vi "cummulative_threshold.vi"(0 "N":dbl[](array[numeric]), 5 "q(i)":dbl[](array[numeric]), 7 "Array 1 in":dbl[](array[numeric]), 9 "Array 2 in":dbl[](array[numeric]), 11 "Array 3 in":dbl[](array[numeric])) -> (4 "Cummulative Threshold Estimate [dB]":dbl=19.38227816273107, 8 "Array 1 out":dbl[](array[numeric]), 10 "Array 2 out":dbl[](array[numeric]), 15 "Array 3 out":dbl[](array[numeric]))   [LabVIEW 2022 SP3]
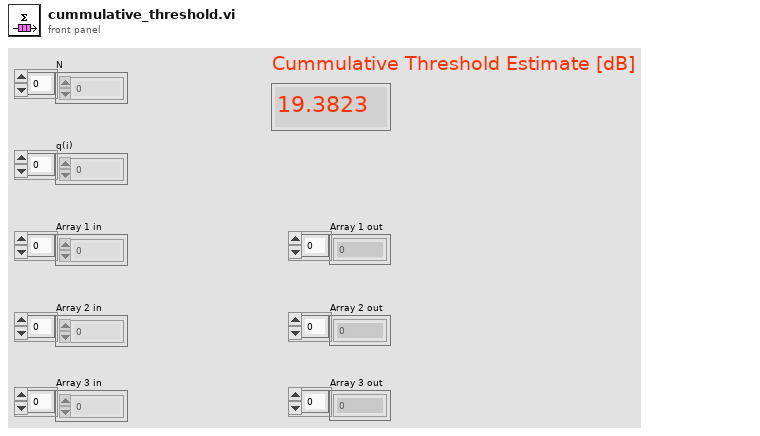
[diagram p1: front panel]
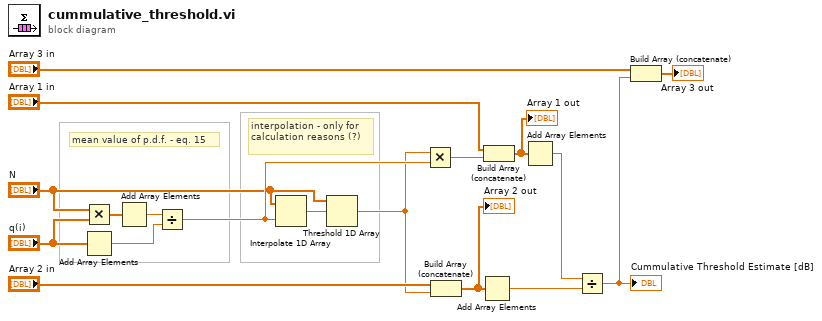
[diagram p0: block diagram]
diagram:
  # "interpolation - only for calculation reasons (?)"
  # "mean value of p.d.f. - eq. 15"
  n1 = Multiply(x="N", y="q(i)") -> (x*y=w3:dbl[])
  n2 = Add Array Elements(numeric array="q(i)") -> (sum=w18:dbl)
  n3 = Add Array Elements(numeric array=w3) -> (sum=w4:dbl)
  n4 = Divide(x=w4, y=w18) -> (x/y=w16:dbl)
  n5 = Interpolate 1D Array(1:w16, 2:"N") -> (0:w17:dbl)
  n6 = Threshold 1D Array(2:w17, 3:"N") -> (0:w8:dbl)  [unwired: 1 in]
  n7 = Multiply(x=w8, y=w16) -> (x*y=w15:dbl)
  n8 = Build Array (concatenate)("Array 2 in", w8) -> (w6:dbl[])
  "Array 2 out" <- w6
  n9 = Add Array Elements(numeric array=w6) -> (sum=w11:dbl)
  n10 = Build Array (concatenate)("Array 1 in", w15) -> (w5:dbl[])
  "Array 1 out" <- w5
  n11 = Add Array Elements(numeric array=w5) -> (sum=w12:dbl)
  n12 = Divide(x=w12, y=w11) -> (x/y=w9:dbl)
  "Cummulative Threshold Estimate [dB]" <- w9
  n13 = Build Array (concatenate)("Array 3 in", w9) -> (→"Array 3 out":dbl[])
